vi "R5SBRControl.vi"(8 "error constant":errorcluster, 11 "LabVIEW Web Service":refnum<class "Web Service.lvclass">) -> (0 "error out":errorcluster)   [LabVIEW 2016]
uses:
  <vilib>/wsapi/Web Service.lvclass
  <vilib>/Platform/TimedLoop/XDataNode/timing_clust.ctl
  <vilib>/Platform/TimedLoop/XDataNode/nitl_modes.ctl
  <vilib>/Platform/TimedLoop/XDataNode/wakeup.ctl
  <vilib>/Platform/TimedLoop/XDataNode/loadnilvce.vi
  <vilib>/Platform/TimedLoop/XDataNode/XDataNode.xnode
  <vilib>/Utility/Variable/NI_VariableUtilities.lvlib
  <vilib>/Platform/TimedLoop/XDataNode/XDNodeRunTimeDep.lvlib
panel:
  out "Numeric 2":i32
  out "current time":timestamp
  out "No phases":i32
  out "Numeric":i32
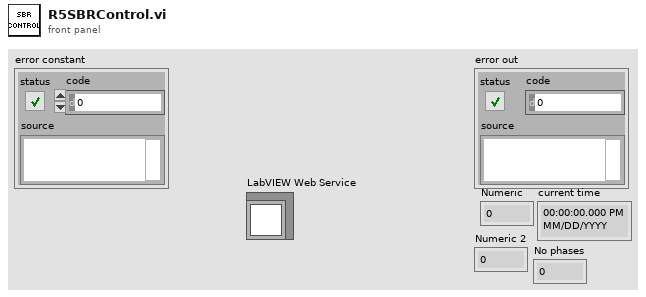
[diagram p1: front panel]
types:
  T1 = typedef "XDNodeRunTimeDep.lvlib/timing_clust.ctl" = cluster{"Expected End [f-1]":u64, "Actual End [f-1]":u64, "Finished Late? [f-1]":bool, "Expected End [i-1]":u64, "Actual End [i-1]":u64, "Finished Late? [i-1]":bool, "Expected Start [i]":u64, "Actual Start [i]":u64, "Expected Start [f]":u64, "Actual Start [f]":u64, "Source Name":string, "Structure Name":string, "Period":i64, "Deadline":i64, "Offset":i64, "Start":i64, "Priority":i32, "Timeout":i32, "Mode":T2, "Wakeup Reason":T3, "Error":errorcluster, "Source Type":string, "Secondary Source Type":string, "Global End Time":u64, "Global Start Time":u64, "Frame Duration":u64, "Iteration Duration":u64, "Assigned CPU":i32, "I/O Scan Engine Mode":u32}
  T2 = typedef "XDNodeRunTimeDep.lvlib/nitl_modes.ctl" = enum32{"No Change", "Process missed periods, maintain original phase", "Discard missed periods, maintain original phase", "Process missed periods, ignore original phase", "Discard missed periods, ignore original phase"}
  T3 = typedef "XDNodeRunTimeDep.lvlib/wakeup.ctl" = enum32{"Normal", "Aborted", "Asynchronous wakeup", "Timing source error", "Timed loop error", "Timeout"}
  T4 = cluster{"Phase":string, "Time, min":dbl, "SBR_Manual":cluster{"Influent Pump":bool, "Effluent Pump":bool}}[]
  T5 = cluster{"Influent Pump":bool, "Effluent Pump":bool}
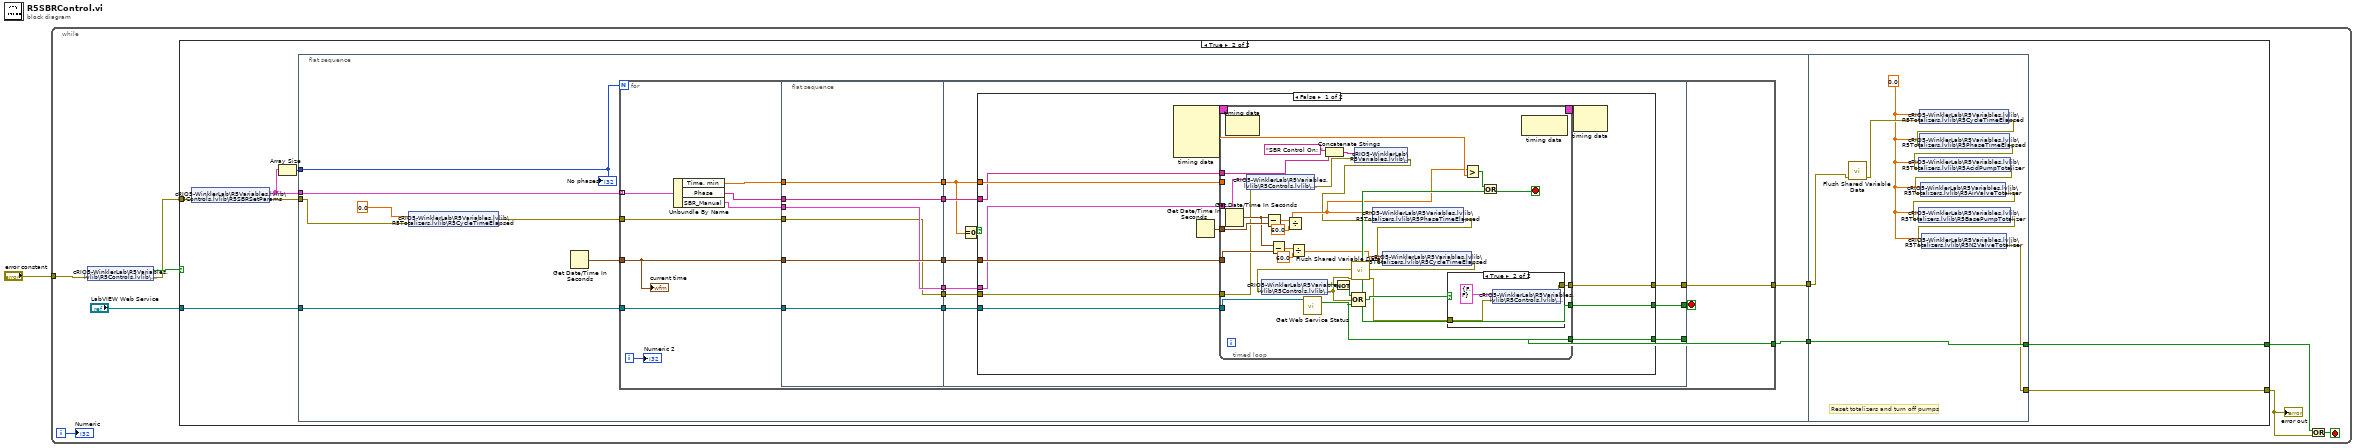
[diagram p0: block diagram]
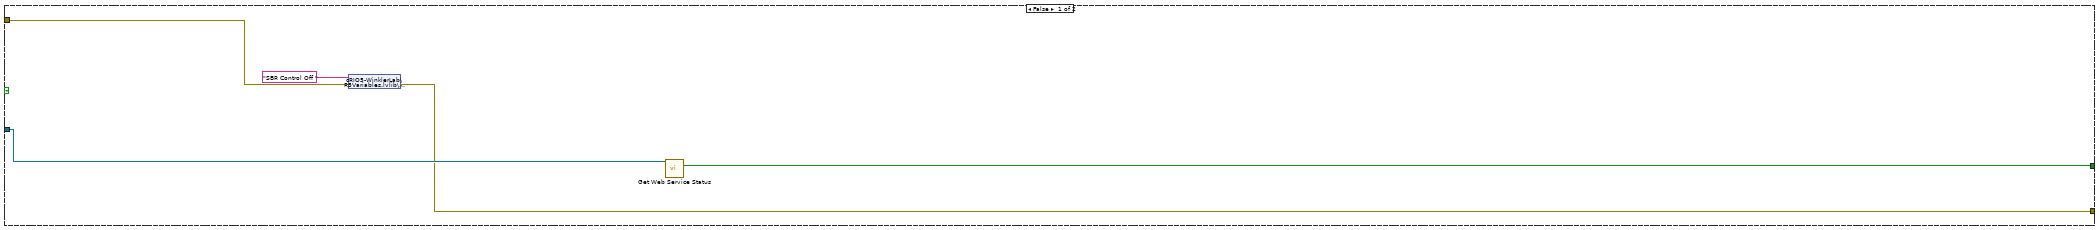
[diagram p2: hidden frame]
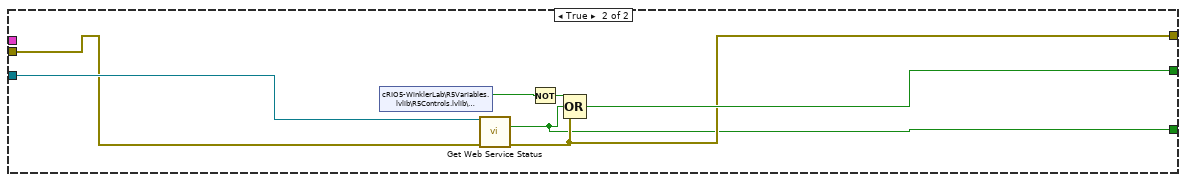
[diagram p4: hidden frame]
diagram:
  n1 = while {
    tunnel: "error constant" -> [w3]
    i -> [w6]
    stop <- w7 stop-if-true
    n2 = shared-variable "cRIO5-WinklerLab\\R5Variables.lvlib\\R5Controls.lvlib\\R5SBRSwitch"(error in=w3) -> (w4:bool, error out=w2:errorcluster)
    n3 = case shown="True" w4 {
      tunnel: "LabVIEW Web Service" -> [w14 w22]
      tunnel: w2 -> [w11 w15]
      tunnel: [w10 w18] -> w8
      tunnel: [w13 w20] -> w5
      frame False {
        n4 = shared-variable "cRIO5-WinklerLab\\R5Variables.lvlib\\R5Status"("SBR Control Off " ("string"), error in=w11) -> (error out=w10:errorcluster)
        n5 = call <vilib>:"Get Web Service Status.vi"("LabVIEW Web Service"=w14) -> ("service stopping?"=w13:bool)  [unwired: 12 in, 2 out]
      }
      frame True {
        n6 = shared-variable "cRIO5-WinklerLab\\R5Variables.lvlib\\R5Controls.lvlib\\R5SBRSetParams"(error in=w15) -> (w17:T4, error out=w16:errorcluster)
        n7 = Array Size(array=w17) -> (size(s)=w23:i32)
        n8 = flat-sequence {
          tunnel: w17 -> [w31]
          tunnel: w23 -> [w32]
          tunnel: w22 -> [w30]
          tunnel: w16 -> [w25]
          tunnel: [w28] -> w21
          tunnel: [w27] -> w19
          tunnel: w21 -> [w131]
          tunnel: [w130] -> w20
          tunnel: w19 -> [w130]
          tunnel: [w127] -> w18
          frame #0 {
            n9 = shared-variable "cRIO5-WinklerLab\\R5Variables.lvlib\\R5Totalizers.lvlib\\R5CycleTimeElapsed"(0.0 ("R1CycleTimeElapsed"), error in=w25) -> (error out=w26:errorcluster)
            n10 = Get Date/Time In Seconds() -> (seconds since 1Jan1904=w29:timestamp)
            n11 = for {
              N: w32 -> [_]
              tunnel: w31 -> [w49] mode=indexing
              tunnel: w30 -> [w47]
              tunnel: w26 -> [w41]
              tunnel: [w39] -> w28
              tunnel: w29 -> [w36]
              tunnel: [w35] -> w27
              i -> [w37]
              stop <- w38 stop-if-true
              n12 = Unbundle By Name(w49) -> ("Time, min"=w44:dbl, "Phase"=w43:string, "SBR_Manual"=w48:T5)
              n13 = flat-sequence {
                tunnel: w44 -> [w54]
                tunnel: w48 -> [w51]
                tunnel: w47 -> [w55]
                tunnel: [w55] -> w46
                tunnel: [w54] -> w45
                tunnel: w43 -> [w53]
                tunnel: [w53] -> w42
                tunnel: w41 -> [w50]
                tunnel: w36 -> [w52]
                tunnel: [w52] -> w40
                tunnel: [w51] -> w34
                tunnel: [w50] -> w33
                tunnel: [w64] -> w38
                tunnel: w46 -> [w65]
                tunnel: w45 -> [w56]
                tunnel: w42 -> [w63]
                tunnel: w40 -> [w62]
                tunnel: [w61] -> w39
                tunnel: [w60] -> w35
                tunnel: w34 -> [w59]
                tunnel: w33 -> [w58]
                frame #0 {
                }
                frame #1 {
                  n14 = Equal To 0?(x=w56) -> (x = 0?=w57:bool)
                  n15 = case shown="False" w57 {
                    tunnel: w65 -> [w77 w120]
                    tunnel: [w76 w118] -> w64
                    tunnel: w63 -> [w66 _]
                    tunnel: w62 -> [w74 _]
                    tunnel: [w73 w117] -> w61
                    tunnel: [w72 w116] -> w60
                    tunnel: w59 -> [w67 _]
                    tunnel: w58 -> [w68 w119]
                    tunnel: w56 -> [w71 _]
                    frame False {
                      n16 = node-c288() -> (w70:T1)  [unwired: 4 in]
                      n17 = Get Date/Time In Seconds() -> (seconds since 1Jan1904=w75:timestamp)
                      n18 = timed-loop {
                        tunnel: w77 -> [w100]
                        tunnel: [w96] -> w76
                        tunnel: w75 -> [w104]
                        tunnel: w74 -> [w101]
                        tunnel: [w94] -> w73
                        tunnel: [w97] -> w72
                        tunnel: w68 -> [w82]
                        tunnel: w71 -> [w93]
                        timing: w70 -> [_]
                        timing-out: [_] -> w69
                        tunnel: w67 -> [w78]
                        tunnel: w66 -> [w89]
                        stop <- w92 stop-if-true
                        n19 = node-c288() -> ()  [unwired: 1 in, 1 out]
                        n20 = Get Date/Time In Seconds() -> (seconds since 1Jan1904=w102:timestamp)
                        n21 = shared-variable "cRIO5-WinklerLab\\R5Variables.lvlib\\R5Controls.lvlib\\R5SBRManual"(w78, error in=w82) -> (error out=w83:errorcluster)
                        n22 = Subtract(x=w102, y=w104) -> (x-y=w105:dbl)
                        n23 = Subtract(x=w102, y=w101) -> (x-y=w99:dbl)
                        n24 = Divide(x=w105, y=60.0) -> (x/y=w85:dbl)
                        n25 = Divide(x=w99, y=60.0) -> (x/y=w87:dbl)
                        n26 = call <vilib>:"Get Web Service Status.vi"("LabVIEW Web Service"=w100) -> ("service stopping?"=w97:bool)  [unwired: 12 in, 2 out]
                        n27 = Concatenate Strings("SBR Control On: " ("string"), w89) -> (w88:string)
                        n28 = shared-variable "cRIO5-WinklerLab\\R5Variables.lvlib\\R5Status"(w88, error in=w83) -> (error out=w84:errorcluster)
                        n29 = shared-variable "cRIO5-WinklerLab\\R5Variables.lvlib\\R5Totalizers.lvlib\\R5PhaseTimeElapsed"(w85, error in=w84) -> (error out=w86:errorcluster)
                        n30 = shared-variable "cRIO5-WinklerLab\\R5Variables.lvlib\\R5Totalizers.lvlib\\R5CycleTimeElapsed"(w87, error in=w86) -> (error out=w79:errorcluster)
                        n31 = shared-variable "cRIO5-WinklerLab\\R5Variables.lvlib\\R5Controls.lvlib\\R5SBRSwitch"(error in=w79) -> (w81:bool, error out=w80:errorcluster)
                        n32 = Not(x=w81) -> (.not. x?=w106:bool)
                        n33 = call <vilib>:"Flush Shared Variable Data.vi"("error in (no error)"=w80) -> ("error out"=w95:errorcluster)  [unwired: 10 in]
                        n34 = Compound Arithmetic op=OR(w106, w80, w97) -> (w96:bool)
                        n35 = case shown="True" w96 {
                          tunnel: w95 -> [w109 w110]
                          tunnel: [w109 w112] -> w94
                          frame False {
                          }
                          frame True {
                            n36 = shared-variable "cRIO5-WinklerLab\\R5Variables.lvlib\\R5Controls.lvlib\\R5SBRManual"(cluster{"Media Pump":bool, "Effluent Pump":bool} {"Media Pump"=FALSE, "Effluent Pump"=FALSE} ("R5SBRManual"), error in=w110) -> (error out=w112:errorcluster)
                          }
                        }
                        n37 = Greater?(x=w85, y=w93) -> (0:w91:bool)
                        n38 = Or(x=w91, y=w96) -> (x .or. y?=w92:bool)
                        n39 = node-c288() -> ()  [unwired: 1 in, 1 out]
                      }
                      n40 = node-c288(w69) -> ()  [unwired: 1 out]
                    }
                    frame True {
                      n41 = shared-variable "cRIO5-WinklerLab\\R5Variables.lvlib\\R5Controls.lvlib\\R5SBRSwitch"() -> (w115:bool)  [unwired: 1 in, 1 out]
                      n42 = call <vilib>:"Get Web Service Status.vi"("LabVIEW Web Service"=w120, "error in (no error)"=w119) -> ("service stopping?"=w116:bool, "error out"=w117:errorcluster)  [unwired: 11 in, 1 out]
                      n43 = Not(x=w115) -> (.not. x?=w121:bool)
                      n44 = Compound Arithmetic op=OR(w121, w116, w117) -> (w118:bool)
                    }
                  }
                }
              }
              "Numeric 2" <- w37
              "current time" <- w36
            }
            "No phases" <- w32
          }
          frame #1 {
            w126 = 0.0 ("R1CycleTimeElapsed")
            # "Reset totalizers and turn off pumps"
            n45 = call <vilib>:"Flush Shared Variable Data.vi"("error in (no error)"=w131) -> ("error out"=w128:errorcluster)  [unwired: 10 in]
            n46 = shared-variable "cRIO5-WinklerLab\\R5Variables.lvlib\\R5Totalizers.lvlib\\R5CycleTimeElapsed"(w126, error in=w128) -> (error out=w129:errorcluster)
            n47 = shared-variable "cRIO5-WinklerLab\\R5Variables.lvlib\\R5Totalizers.lvlib\\R5PhaseTimeElapsed"(w126, error in=w129) -> (error out=w125:errorcluster)
            n48 = shared-variable "cRIO5-WinklerLab\\R5Variables.lvlib\\R5Totalizers.lvlib\\R5AcidPumpTotalizer"(w126, error in=w125) -> (error out=w124:errorcluster)
            n49 = shared-variable "cRIO5-WinklerLab\\R5Variables.lvlib\\R5Totalizers.lvlib\\R5AirValveTotalizer"(w126, error in=w124) -> (error out=w123:errorcluster)
            n50 = shared-variable "cRIO5-WinklerLab\\R5Variables.lvlib\\R5Totalizers.lvlib\\R5BasePumpTotalizer"(w126, error in=w123) -> (error out=w122:errorcluster)
            n51 = shared-variable "cRIO5-WinklerLab\\R5Variables.lvlib\\R5Totalizers.lvlib\\R5N2ValveTotalizer"(w126, error in=w122) -> (error out=w127:errorcluster)
          }
        }
      }
    }
    "error out" <- w8
    n52 = Or(x=w5, y=w8) -> (x .or. y?=w7:bool)
    "Numeric" <- w6
  }
